vi "FireMotor.vi"   [LabVIEW 2012]
uses:
  StateMachineEnum.ctl
  Robot Global Data.vi
types:
  T1 = typedef "StateMachineEnum.ctl" = enum16{"Init", "Idle", "Start", "Do", "Stop"}
  T2 = typedef "WPI_MotorControlDeviceRef.ctl" = cluster{"DeviceStatus":errorcluster, "Type":enum16{"PWM", "CAN"}, "PWM":cluster{"Digital Module":T3, "PWM Channel":T4, "DeadBand":T5}, "CAN":cluster{"Device Number":u8, "Control Mode":T6, "Semaphore":T7, "Max Vout":dbl}, "Invert":bool, "TransformRef":T8, "InvTransformRef":T8}
  T3 = typedef "FPGA_TypedefDigitalModule.ctl" = enum16{"Digital Module 1", "Digital Module 2"}
  T4 = typedef "FPGA_DIOPWMChannel.ctl" = enum8{"PWM 1", "PWM 2", "PWM 3", "PWM 4", "PWM 5", "PWM 6", "PWM 7", "PWM 8", "PWM 9", "PWM 10", "Invalid"}
  T5 = typedef "WPI_PWMDeadband.ctl" = cluster{"Name":string, "maxPositivePwm":i32, "minPositivePwm":i32, "centerPwm":i32, "maxNegativePwm":i32, "minNegativePwm":i32, "angularRange":u16}
  T6 = typedef "WPI_CANJaguar_ControlMode.ctl" = enum8{"Percent VBus", "Current", "Speed", "Position", "Voltage"}
  T7 = typedef "Semaphore RefNum" = refnum<k1>
  T8 = typedef "WPI_PWMTransform_ConPane.ctl" = refnum<vi>
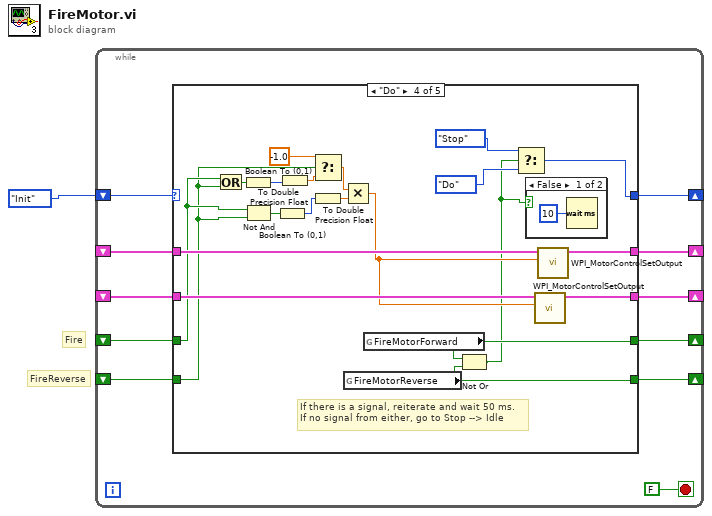
[diagram p0: block diagram]
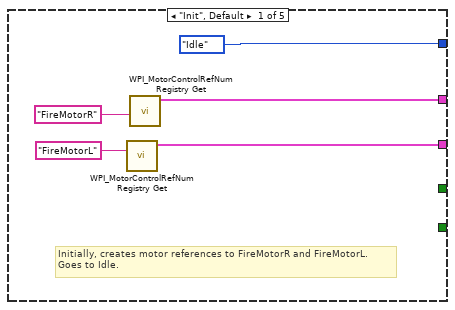
[diagram p2: hidden frame]
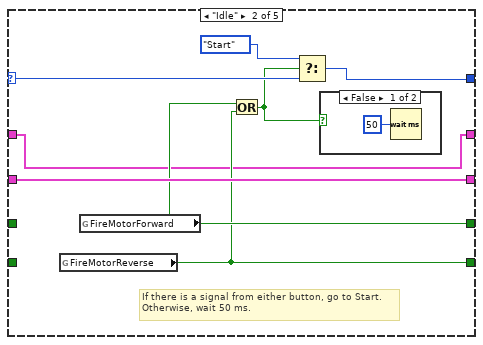
[diagram p3: hidden frame]
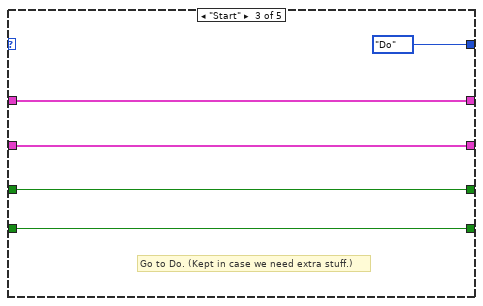
[diagram p5: hidden frame]
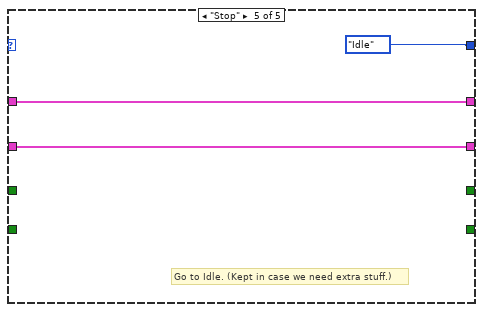
[diagram p7: hidden frame]
diagram:
  # "FireReverse"
  # "Fire"
  n1 = while {
    shift-right: [w2] -> _
    shift-left: StateMachineEnum."Init" ("State") -> [w7]
    shift-right: [w12] -> _
    shift-left: _ -> [w9]
    shift-right: [w11] -> _
    shift-left: _ -> [w8]
    shift-right: [w5] -> _
    shift-left: _ -> [w3]
    shift-right: [w6] -> _
    shift-left: _ -> [w4]
    stop <- FALSE stop-if-true
    n2 = case shown="\"Do\"" w7 {
      selector: w7 -> [_ w23 _ _ _]
      tunnel: [StateMachineEnum."Idle" ("State") w19 StateMachineEnum."Do" ("State") w46 StateMachineEnum."Idle" ("State")] -> w2
      tunnel: [w14 w20 w30 w49 w56] -> w12
      tunnel: [w13 w24 w29 w51 w55] -> w11
      tunnel: w9 -> [_ w20 w30 w50 w56]
      tunnel: w8 -> [_ w24 w29 w52 w55]
      tunnel: [_ w21 w27 w33 _] -> w6
      tunnel: [_ w22 w28 w34 _] -> w5
      tunnel: w4 -> [_ _ w27 w42 _]
      tunnel: w3 -> [_ _ w28 w43 _]
      frame "Init", Default {
        # "Initially, creates motor references to FireMotorR and FireMotorL.\nGoes to Idle."
        n3 = call <vilib>:"WPI_MotorControlRefNum Registry Get.vi"("refnum name"="FireMotorL") -> ("MotorControlDevRef"=w13:T2)  [unwired: 9 in, 1 out]
        n4 = call <vilib>:"WPI_MotorControlRefNum Registry Get.vi"("refnum name"="FireMotorR") -> ("MotorControlDevRef"=w14:T2)  [unwired: 9 in, 1 out]
      }
      frame "Idle" {
        # "If there is a signal from either button, go to Start.\nOtherwise, wait 50 ms."
        n5 = global read "Robot Global Data.vi" "FireMotorReverse"() -> (w21:bool)
        n6 = global read "Robot Global Data.vi" "FireMotorForward"() -> (w22:bool)
        n7 = Or(x=w22, y=w21) -> (x .or. y?=w18:bool)
        n8 = Select(t=StateMachineEnum."Start" ("State"), s=w18, f=w23) -> (s? t:f=w19:T1)
        n9 = case shown="False" w18 {
          frame False {
            n10 = Wait (ms)(milliseconds to wait=u32 50) -> ()  [unwired: 1 out]
          }
          frame True {
          }
        }
      }
      frame "Start" {
        # "Go to Do. (Kept in case we need extra stuff.)"
      }
      frame "Do" {
        # "If there is a signal, reiterate and wait 50 ms.\nIf no signal from either, go to Stop --> Idle"
        n11 = Or(x=w43, y=w42) -> (x .or. y?=w45:bool)
        n12 = Boolean To (0,1)(Boolean=w45) -> (0, 1=w44:i16)
        n13 = Not And(1:w42, 2:w43) -> (0:w41:bool)
        n14 = Boolean To (0,1)(Boolean=w41) -> (0, 1=w39:i16)
        n15 = To Double Precision Float(number=w44) -> (double precision float=w36:dbl)
        n16 = Select(t=-1.0, s=w42, f=w36) -> (s? t:f=w40:dbl)
        n17 = To Double Precision Float(number=w39) -> (double precision float=w37:dbl)
        n18 = Multiply(x=w40, y=w37) -> (x*y=w38:dbl)
        n19 = global read "Robot Global Data.vi" "FireMotorReverse"() -> (w33:bool)
        n20 = global read "Robot Global Data.vi" "FireMotorForward"() -> (w34:bool)
        n21 = Not Or(1:w33, 2:w34) -> (0:w32:bool)
        n22 = Select(t=StateMachineEnum."Stop" ("State"), s=w32, f=StateMachineEnum."Do" ("State")) -> (s? t:f=w46:T1)
        n23 = case shown="False" w32 {
          frame False {
            n24 = Wait (ms)(milliseconds to wait=u32 10) -> ()  [unwired: 1 out]
          }
          frame True {
          }
        }
        n25 = call <vilib>:"WPI_MotorControlSetOutput.vi"("Output"=w38, "MotorControlDevRef"=w52) -> ("MotorControlDevRef"=w51:T2)  [unwired: 7 in, 2 out]
        n26 = call <vilib>:"WPI_MotorControlSetOutput.vi"("Output"=w38, "MotorControlDevRef"=w50) -> ("MotorControlDevRef"=w49:T2)  [unwired: 7 in, 2 out]
      }
      frame "Stop" {
        # "Go to Idle. (Kept in case we need extra stuff.)"
      }
    }
  }
